vi "DeviceDiscovery.vi"(4 "error in (no error)":errorcluster, 7 "logging":bool) -> (0 "error out":errorcluster, 2 "CmdLib Out":refnum<k24>, 3 "VCPIOLib Out":refnum<k24>)   [LabVIEW 2013]
uses:
  C:/Code/Apps/Utilities/AG-UC2-UC8/AG-UC2-UC8/Install/Samples/LabVIEW/LabVIEW 2013/VCPIOLib.dll
  VCPIOLib.dll
  C:/Code/Apps/Utilities/AG-UC2-UC8/AG-UC2-UC8/Install/Samples/LabVIEW/LabVIEW 2013/CmdLibAgilis.dll
  CmdLibAgilis.dll
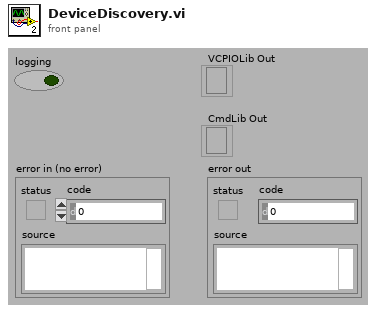
[diagram p1: front panel]
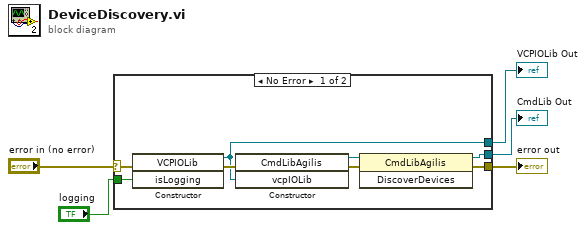
[diagram p0: block diagram]
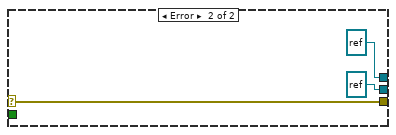
[diagram p2: hidden frame]
diagram:
  n1 = case shown="No Error" "error in (no error)" {
    selector: "error in (no error)" -> [w11 w16]
    tunnel: "logging" -> [w7 _]
    tunnel: [w13 refnum<k24> refnum ("new reference")] -> w1
    tunnel: [w12 w16] -> w3
    tunnel: [w6 refnum<k24> refnum ("new reference")] -> w2
    frame No Error {
      n2 = constructor class="VCPIOLib"(error in=w11, "isLogging"=w7) -> (reference out=w6:refnum<k24>, error out=w10:errorcluster)  [unwired: 2 in, 2 out]
      n3 = constructor class="CmdLibAgilis"(error in=w10, "vcpIOLib"=w6) -> (reference out=w8:refnum<k24>, error out=w9:errorcluster)  [unwired: 2 in, 2 out]
      n4 = invoke class="CmdLibAgilis" method="DiscoverDevices"(reference=w8, error in=w9) -> (reference out=w13:refnum<k24>, error out=w12:errorcluster)  [unwired: 1 in, 1 out]
    }
    frame Error {
    }
  }
  "error out" <- w3
  "VCPIOLib Out" <- w2
  "CmdLib Out" <- w1
